vi "svl_Compute Sensor Sensitivity.vi"(8 "channel info in":T1={"sensor sensitivity"=1000.0, "engineering units"=1, "dB reference"=1.0, "custom label"="EU", "weighting filter"=0, "pregain"=0.0} {"pregain" format="%.2f"; "weighting filter" items=["Linear", "A-weighting", "B-weighting", "C-weighting", "ITU-R 468-4", "Dolby", "CCITT", "C-message", "Wb", "Wc", "Wd", "We", "Wf", "Wh", "Wj", "Wk", "Wm", "AES17 20 kHz lowpass", "AES17 40 kHz lowpass", "AES17 20 kHz highpass", "AES17 40 kHz highpass"]; "dB reference" format="%^.1e"; "engineering units" items=["custom..."=0, "V"=1, "A"=21, "C"=30, "pC"=31, "s"=32, "-"=29, "Pa"=2, "N"=20, "g"=3, "m/s^2"=4, "m/s"=5, "m"=6, "mm/s"=12, "mm"=13, "micron/s"=14, "micron"=15, "in/s^2"=7, "in/s"=8, "in"=9, "mil/s"=10, "mil"=11, "rad/s^2"=16, "rad/s"=17, "rad"=18, "deg/s^2"=26, "deg/s"=27, "deg"=28, "RPM"=22, "cycle/s^2"=23, "Hz"=24, "cycle"=25, "strain"=19]; "sensor sensitivity" format="%#_5f"}, 9 "calib. value is in dB (F)":bool, 10 "calibration value [EUrms]":dbl=1.0 format="%.2f", 11 "amplitude (Vrms)":dbl format="%.2f") -> (0 "channel info out":T1={"sensor sensitivity"=1000.0, "engineering units"=1, "dB reference"=1.0, "custom label"="EU", "weighting filter"=0, "pregain"=0.0} {"pregain" format="%.2f"; "weighting filter" items=["Linear", "A-weighting", "B-weighting", "C-weighting", "ITU-R 468-4", "Dolby", "CCITT", "C-message", "Wb", "Wc", "Wd", "We", "Wf", "Wh", "Wj", "Wk", "Wm", "AES17 20 kHz lowpass", "AES17 40 kHz lowpass", "AES17 20 kHz highpass", "AES17 40 kHz highpass"]; "dB reference" format="%^.1e"; "engineering units" items=["custom..."=0, "V"=1, "A"=21, "C"=30, "pC"=31, "s"=32, "-"=29, "Pa"=2, "N"=20, "g"=3, "m/s^2"=4, "m/s"=5, "m"=6, "mm/s"=12, "mm"=13, "micron/s"=14, "micron"=15, "in/s^2"=7, "in/s"=8, "in"=9, "mil/s"=10, "mil"=11, "rad/s^2"=16, "rad/s"=17, "rad"=18, "deg/s^2"=26, "deg/s"=27, "deg"=28, "RPM"=22, "cycle/s^2"=23, "Hz"=24, "cycle"=25, "strain"=19]; "sensor sensitivity" format="%#_5f"}, 3 "sensor sensitivity [mV/EU]":dbl format="%.2f")   [LabVIEW 2017, in "SoundVib_Calibration.lvlib"]
uses:
  <vilib>/addons/Sound and Vibration/svt_Calibration/SoundVib_Calibration.lvlib
  <vilib>/addons/_NISVFA/_Shared subVIs/Controls/svc_Channel Info.ctl
  <vilib>/addons/_NISVFA/_Shared subVIs/Controls/svc_Engineering Units Text Ring.ctl
  <vilib>/addons/_NISVFA/_Shared subVIs/Controls/svc_Weighting Filter Text Ring.ctl
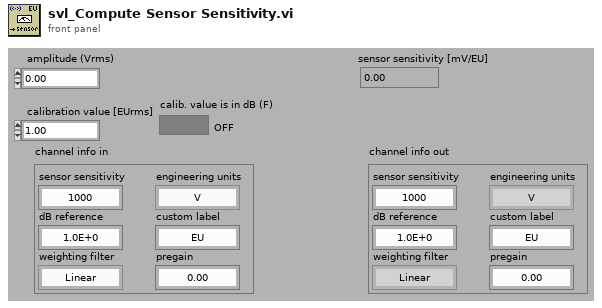
[diagram p1: front panel]
types:
  T1 = typedef "svc_Channel Info.ctl" = cluster{"sensor sensitivity":dbl, "engineering units":T2, "dB reference":dbl, "custom label":string, "weighting filter":T3, "pregain":dbl}
  T2 = typedef "svc_Engineering Units Text Ring.ctl" = u16
  T3 = typedef "svc_Weighting Filter Text Ring.ctl" = u16
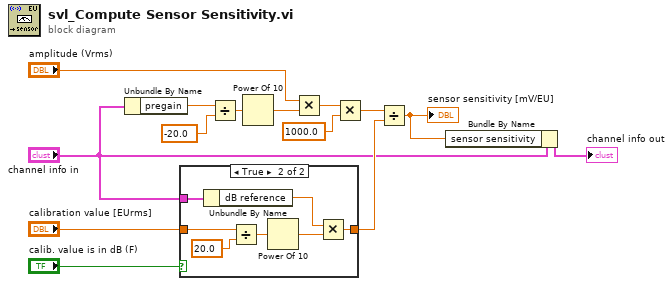
[diagram p0: block diagram]
diagram:
  n1 = Unbundle By Name("channel info in") -> ("pregain"=w14:dbl)
  n2 = case shown="True" "calib. value is in dB (F)" {
    tunnel: "calibration value [EUrms]" -> [w15 w22]
    tunnel: [w15 w16] -> w5
    tunnel: "channel info in" -> [_ w19]
    frame False {
    }
    frame True {
      n3 = Unbundle By Name(w19) -> ("dB reference"=w17:dbl)
      n4 = Divide(x=w22, y=20.0) -> (x/y=w20:dbl)
      n5 = Power Of 10(x=w20) -> (10^x=w18:dbl)
      n6 = Multiply(x=w17, y=w18) -> (x*y=w16:dbl)
    }
  }
  n7 = Divide(x=w14, y=-20.0) -> (x/y=w12:dbl)
  n8 = Power Of 10(x=w12) -> (10^x=w11:dbl)
  n9 = Multiply(x="amplitude (Vrms)", y=w11) -> (x*y=w10:dbl)
  n10 = Multiply(x=w10, y=1000.0) -> (x*y=w8:dbl)
  n11 = Divide(x=w8, y=w5) -> (x/y=w1:dbl)
  "sensor sensitivity [mV/EU]" <- w1
  n12 = Bundle By Name(cluster="channel info in", "sensor sensitivity"=w1) -> (→"channel info out":T1)
